vi "Load IOPanel.vi"(8 "error in (no error)":errorcluster, 11 "MPC_Laser Marked in":refnum<class "MPC_Laser Marked.lvclass">) -> (0 "error out":errorcluster, 2 "This VI":refnum<vi>, 3 "MPC_Laser Marked out":refnum<class "MPC_Laser Marked.lvclass">)   [LabVIEW 2019, in "MPC_Laser Marked.lvclass"]
uses:
  MPC_Laser Marked.lvclass
  <vilib>/Utility/miscctls.llb/LVPositionTypeDef.ctl
  Function/IO Folder/IO_VI/IOCtrl/Ctrl/IO Card_Type.ctl
  Function/IO Folder/IO_Class/IOCard.lvclass
  Function/IO Folder/IO_Class/IOCard.lvclass/IOCard.ctl
panel:
  in  "Tab Control":enum32{"Page 1", "Page 2"}(tab)
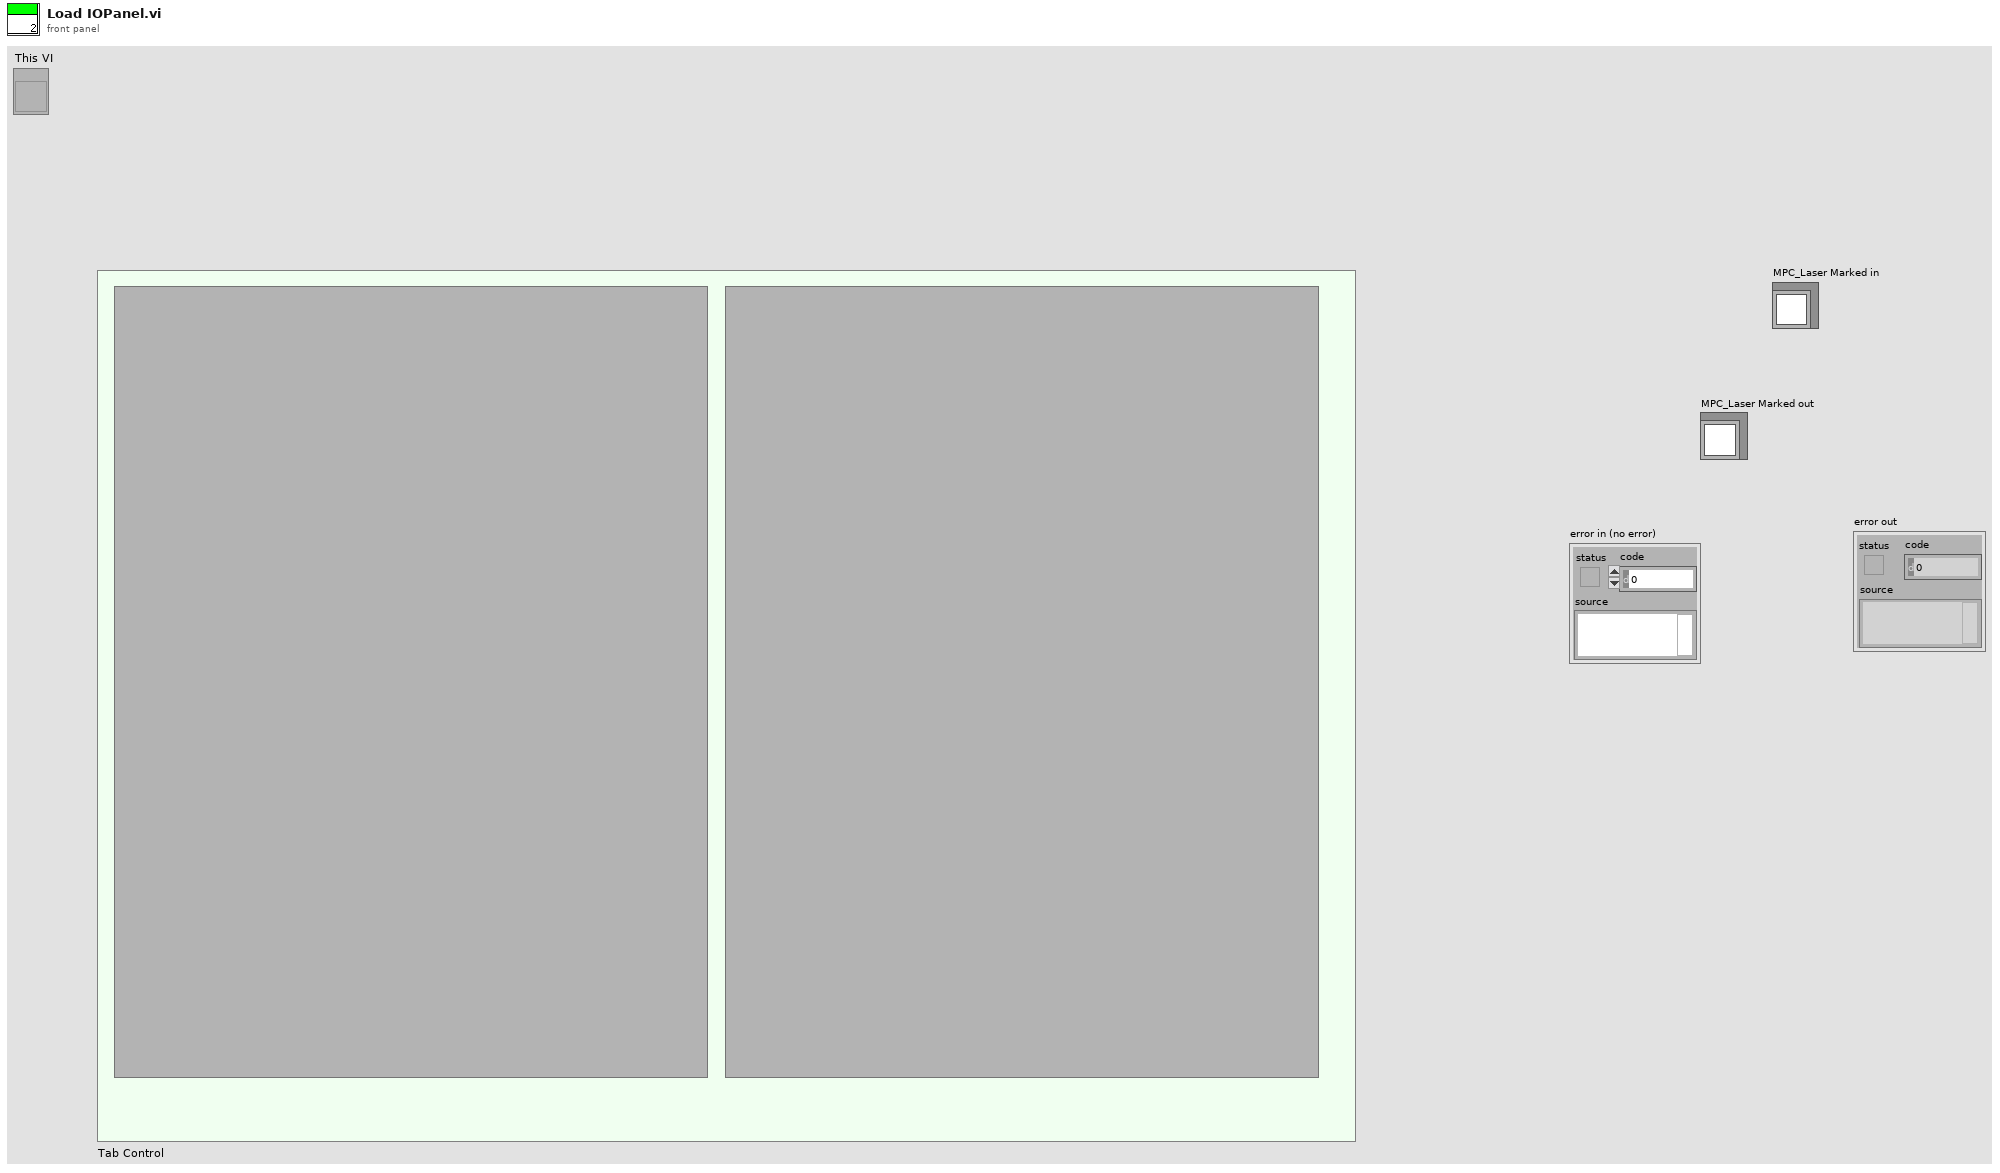
[diagram p1: front panel]
types:
  T1 = typedef "LVPositionTypeDef.ctl" = cluster{"Left":i32, "Top":i32}
  T2 = typedef "IO Card_Type.ctl" = enum16{"None", "Unidaq32", "6480", "2410C-64", "Zan", "DMC1000B", "16InOut", "Robot", "DMC3600"}
  T3 = cluster{"IO Card Type":T2, "IOType":enum16{"Input", "Output"}, "CardNumber":i32, "ConnectAct":bool, "IP":string}
  T4 = typedef "LVPointTypeDef.ctl" = cluster{"Horizontal":i16, "Vertical":i16}
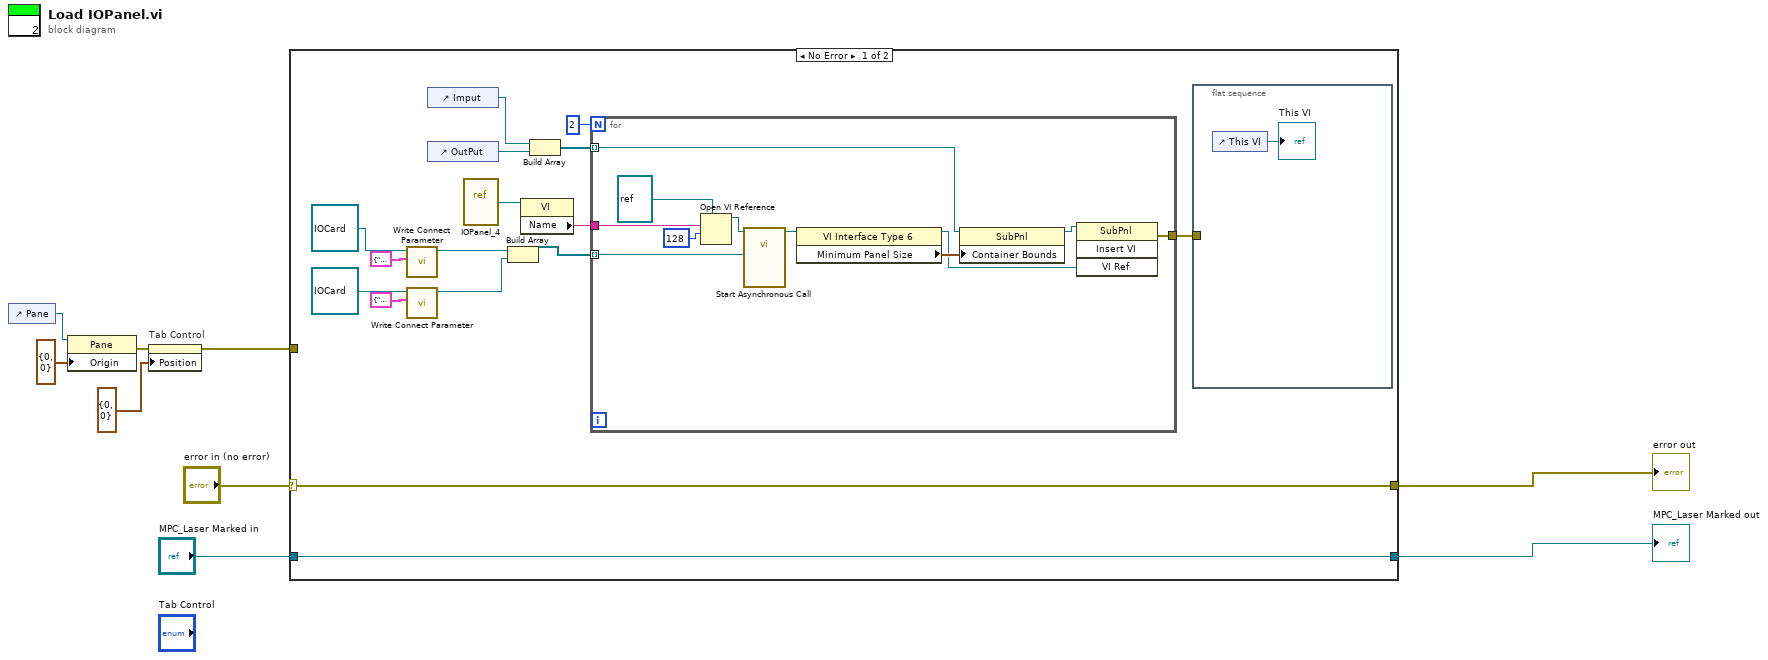
[diagram p0: block diagram]
diagram:
  n1 = control-ref of="Pane"() -> (w5:refnum<vi>)
  n2 = property class="Pane"(reference=w5, "Origin"=T1 {"Left"=0, "Top"=0} ("Position")) -> (error out=w4:errorcluster)  [unwired: 1 in, 1 out]
  n3 = property on="Tab Control" class="TabCtl (strict)"(error in=w4, "Position"=T1 {"Left"=0, "Top"=0}) -> (error out=w1:errorcluster)  [unwired: 1 in, 1 out]
  n4 = case shown="No Error" "error in (no error)" {
    selector: "error in (no error)" -> [w17 w39]
    tunnel: [w17 w39] -> w8
    tunnel: [w16 w38] -> w7
    tunnel: "MPC_Laser Marked in" -> [w16 w38]
    tunnel: w1 -> [_ _]
    frame No Error {
      n5 = call "Write Connect Parameter.vi"("Connect Parameter"=T3 {"IO Card Type"=enum."DMC1000B", "IOType"=enum."Input", "CardNumber"=0, "ConnectAct"=TRUE, "IP"=""}, "IOCard in"=refnum<class "IOCard.lvclass"> refnum ("IOCard.lvclass")) -> ("IOCard out"=w14:refnum<class "IOCard.lvclass">)  [unwired: 8 in, 1 out]
      n6 = call "Write Connect Parameter.vi"("Connect Parameter"=T3 {"IO Card Type"=enum."DMC1000B", "IOType"=enum."Output", "CardNumber"=0, "ConnectAct"=FALSE, "IP"=""}, "IOCard in"=refnum<class "IOCard.lvclass"> refnum ("IOCard.lvclass")) -> ("IOCard out"=w12:refnum<class "IOCard.lvclass">)  [unwired: 8 in, 1 out]
      n7 = control-ref of="Imput"() -> (w19:refnum<vi>)
      n8 = control-ref of="OutPut"() -> (w11:refnum<vi>)
      n9 = vi-ref "IOPanel_4.vi"() -> (w10:refnum<vi>)
      n10 = Build Array(w14, w12) -> (w13:refnum<class "IOCard.lvclass">[])
      n11 = property class="VI"(reference=w10) -> ("Name"=w21:string)  [unwired: 1 in, 2 out]
      n12 = Build Array(w19, w11) -> (w18:refnum<vi>[])
      n13 = for {
        N: 2 -> [_]
        tunnel: w21 -> [w37]
        tunnel: w13 -> [w33] mode=indexing
        tunnel: w18 -> [w30] mode=indexing
        tunnel: [w32] -> w15
        n14 = Open VI Reference(type specifier VI Refnum (for type only)=refnum<vi> refnum, vi path=w37, options=128) -> (vi reference=w34:refnum<vi>)  [unwired: 3 in, 1 out]
        n15 = call-by-ref "Start Asynchronous Call"(reference=w34, "IOCard In"=w33) -> (reference out=w31:refnum<vi>)  [unwired: 12 in, 1 out]
        n16 = property class="VI Interface Type 6"(reference=w31) -> (reference out=w27:refnum<vi>, "Minimum Panel Size"=w28:T4)  [unwired: 1 in, 1 out]
        n17 = property class="SubPnl"(reference=w30, "Container Bounds"=w28) -> (reference out=w29:refnum<vi>)  [unwired: 1 in, 1 out]
        n18 = invoke class="SubPnl" method="Insert VI"(reference=w29, "VI Ref"=w27) -> (error out=w32:errorcluster)  [unwired: 2 in, 3 out]
      }
      n19 = flat-sequence {
        tunnel: w15 -> [_]
        frame #0 {
          n20 = control-ref of="This VI"() -> (→"This VI":refnum<vi>)
        }
      }
    }
    frame Error {
    }
  }
  "error out" <- w8
  "MPC_Laser Marked out" <- w7
